vi "solar_voy_def Find Packet (Name).vi"(6 "CMD":enum8{"CMD", "TLM"}(ring), 8 "PACKET":string, 9 "TARGET":string, 10 "PACKETS":T1[](array[typedef]) {"last_time" format="%<%H:%M:%S%3u %m/%d/%y>T"}) -> (2 "Index":i32)   [LabVIEW 2018]
doc: "This searches for a packet by name."
uses:
  solar_voy_def_ctl ITEM TYPE.ctl
  type/solar_type Item Type.ctl
  solar_voy_def_ctl ITEM.ctl
  solar_voy_def_ctl PACKET_ID.ctl
  solar_voy_def_ctl PACKET.ctl
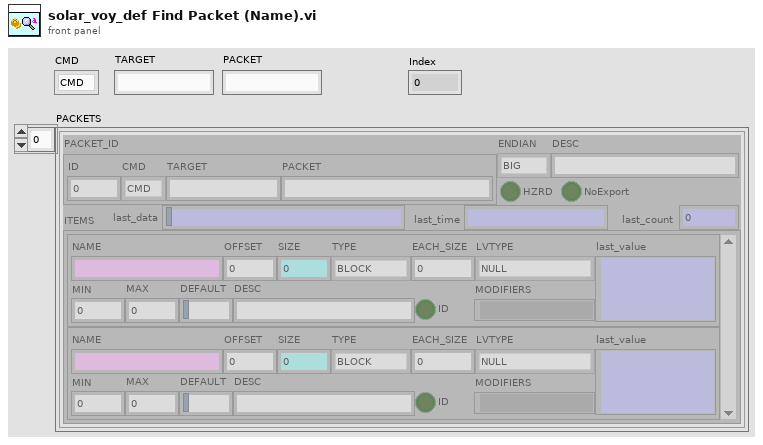
[diagram p1: front panel]
types:
  T1 = typedef "solar_voy_def_ctl PACKET.ctl" = cluster{"PACKET_ID":T2, "ENDIAN":enum8{"BIG", "LITTLE"}, "DESC":string, "HZRD":bool, "ITEMS":T3[], "NoExport":bool, "last_time":timestamp, "last_count":u32, "last_data":string}
  T2 = typedef "solar_voy_def_ctl PACKET_ID.ctl" = cluster{"ID":u16, "CMD":enum8{"CMD", "TLM"}, "TARGET":string, "PACKET":string}
  T3 = typedef "solar_voy_def_ctl ITEM.ctl" = cluster{"NAME":string, "OFFSET":i32, "SIZE":i32, "TYPE":T4, "EACH_SIZE":i32, "LVTYPE":T5, "MIN":dbl, "MAX":dbl, "DEFAULT":string, "DESC":string, "ID":bool, "MODIFIERS":variant, "last_value":variant}
  T4 = typedef "solar_voy_def_ctl ITEM TYPE.ctl" = enum8{"BLOCK", "INT", "UINT", "FLOAT", "STRING"}
  T5 = typedef "solar_type Item Type.ctl" = enum16{"NULL", "UNKNOWN", "CLUSTER", "I8", "I16", "I32", "I64", "U8", "U16", "U32", "U64", "U8_ENUM", "U16_ENUM", "U32_ENUM", "SGL", "DBL", "BOOLEAN", "STRING", "PATH", "VISA", "TAG", "TIME", "I8_1D", "I16_1D", "I32_1D", "I64_1D", "U8_1D", "U16_1D", "U32_1D", "U64_1D", "U8_ENUM_1D", "U16_ENUM_1D", "U32_ENUM_1D", "SGL_1D", "DBL_1D", "BOOLEAN_1D", "STRING_1D", "PATH_1D", "VISA_1D", "TAG_1D", "TIME_1D", "I8_2D", "I16_2D", "I32_2D", "I64_2D", "U8_2D", "U16_2D", "U32_2D", "U64_2D", "U8_ENUM_2D", "U16_ENUM_2D", "U32_ENUM_2D", "SGL_2D", "DBL_2D", "BOOLEAN_2D", "STRING_2D", "PATH_2D", "VISA_2D", "TAG_2D", "TIME_2D"}
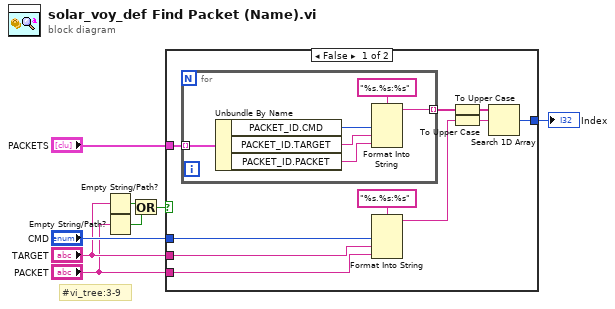
[diagram p0: block diagram]
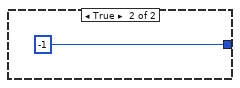
[diagram p2: hidden frame]
diagram:
  # "#vi_tree:3-9"
  n1 = Empty String/Path?(string/path="TARGET") -> (empty?=w3:bool)
  n2 = Empty String/Path?(string/path="PACKET") -> (empty?=w2:bool)
  n3 = Or(x=w3, y=w2) -> (x .or. y?=w1:bool)
  n4 = case shown="False" w1 {
    tunnel: "PACKETS" -> [w18 _]
    tunnel: [w17 -1 ("index of element")] -> w7
    tunnel: "CMD" -> [w13 _]
    tunnel: "TARGET" -> [w12 _]
    tunnel: "PACKET" -> [w11 _]
    frame False {
      n5 = for {
        tunnel: w18 -> [w24] mode=indexing
        tunnel: [w19] -> w16 mode=indexing
        n6 = Unbundle By Name(w24) -> ("PACKET_ID.CMD"=w23:enum8{"CMD", "TLM"}, "PACKET_ID.TARGET"=w22:string, "PACKET_ID.PACKET"=w21:string)
        n7 = Format Into String(format string="%s.%s:%s", w23, w22, w21) -> (resulting string=w19:string)  [unwired: 2 in, 1 out]
      }
      n8 = Format Into String(format string="%s.%s:%s", w13, w12, w11) -> (resulting string=w10:string)  [unwired: 2 in, 1 out]
      n9 = To Upper Case(1:w16) -> (0:w15:string[])
      n10 = To Upper Case(1:w10) -> (0:w9:string)
      n11 = Search 1D Array(1D array=w15, element=w9) -> (index of element=w17:i32)  [unwired: 1 in]
    }
    frame True {
    }
  }
  "Index" <- w7
